vi "Stack_holderwise_total_bd_count_&_duration_2.vi"(0 "Refnum in":T1, 1 "BREAKDOWN_STK_HOLD_ID":i32=1, 2 "condition":string="Where BREAKDOWN_DATE between '%s'and '%s' and BREAKDOWN_STK_HOLD_ID ='%d'  ", 5 "Form Date":timestamp, 7 "Array":string[](array[string]), 9 "To Date":timestamp, 11 "error in (no error)":errorcluster, 12 "STATION_ID_CID_TRIGGER":i32, 13 "Shift":string(combo), 14 "table":string[](array[string])=["STATION_1_LOG_HISTORY", "STATION_2_LOG_HISTORY", "STATION_3_LOG_HISTORY", "STATION_4_LOG_HISTORY", "STATION_5_LOG_HISTORY", "STATION_6_LOG_HISTORY"]) -> (4 "Refnum out":T1, 6 "Count out":string[](array[string]), 10 "appended array":dbl[](array[numeric]), 15 "error out":errorcluster)   [LabVIEW 2017]
uses:
  <vilib>/addons/database/Connection.llb/Conn ObjectReference.ctl
  <vilib>/addons/database/NI_Database_API.lvlib
panel:
  out "Count out 2":string[](array[string])
  out "Table":string[][](array[string])
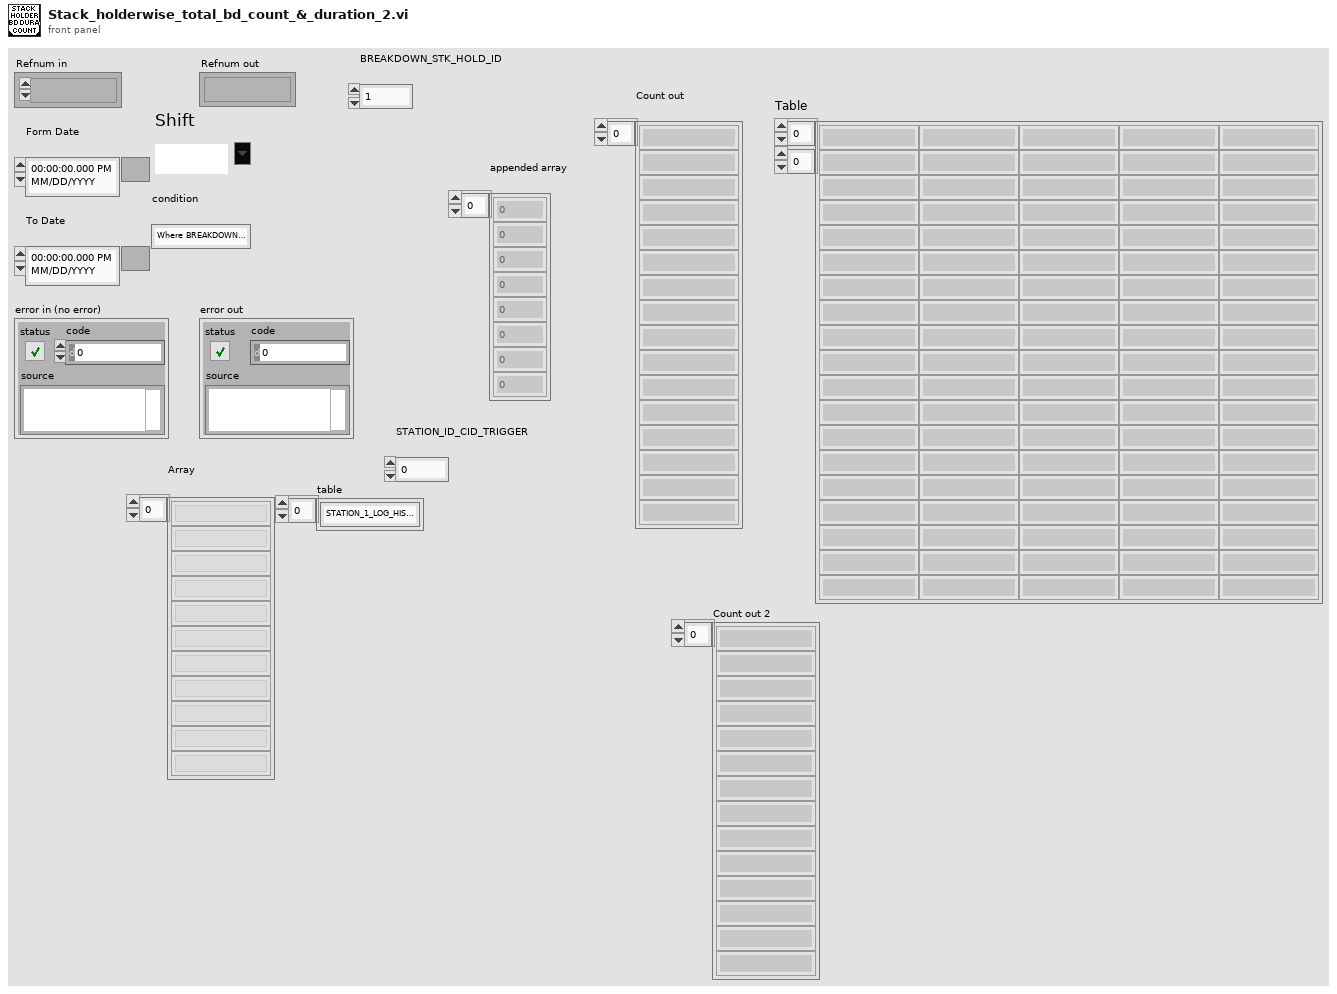
[diagram p1: front panel]
types:
  T1 = typedef "NI_Database_API.lvlib/Conn ObjectReference.ctl" = refnum<k1>
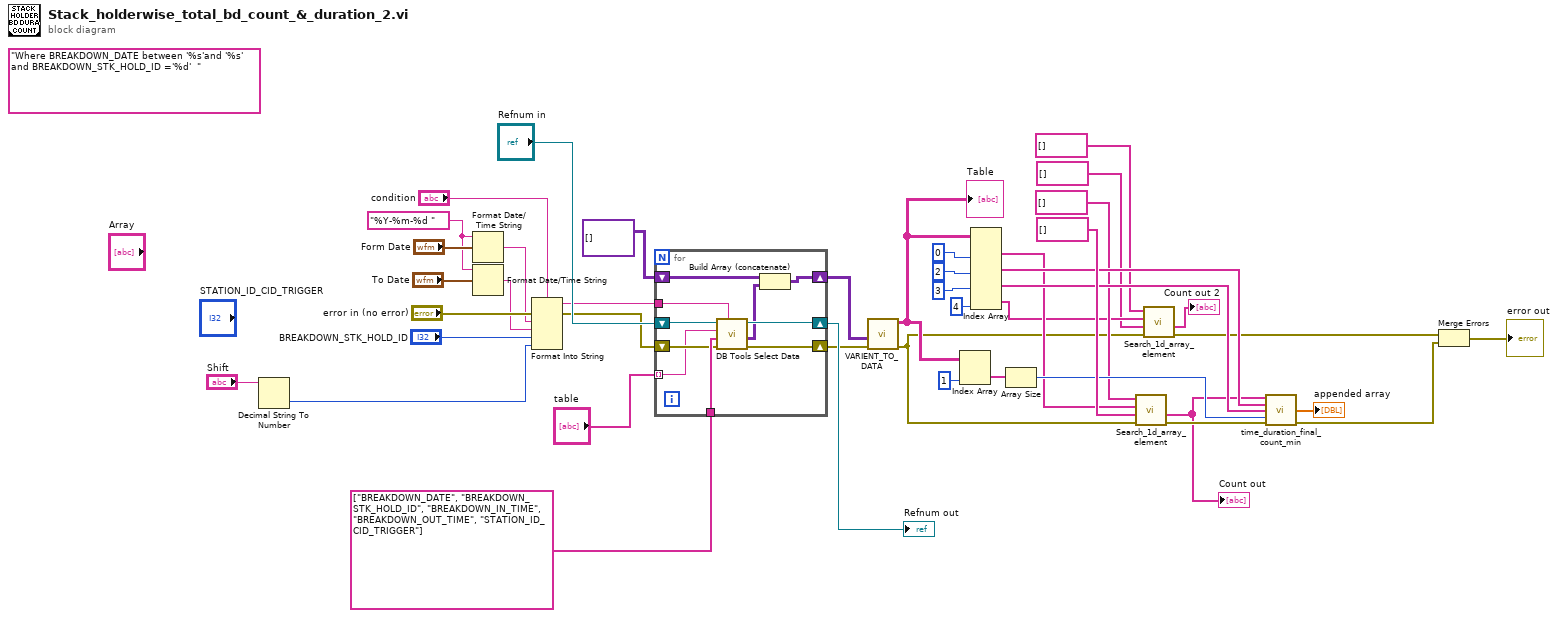
[diagram p0: block diagram]
diagram:
  (unwired) "Where BREAKDOWN_DATE between '%s'and '%s' and BREAKDOWN_STK_HOLD_ID ='%d'  "
  w21 = "%Y-%m-%d " ("time format string (%c)")
  n1 = Decimal String To Number(string="Shift") -> (number=w1:i32)  [unwired: 2 in, 1 out]
  n2 = Format Date/Time String(time format string (%c)=w21, seconds (now)="Form Date") -> (date/time string=w24:string)  [unwired: 1 in]
  n3 = Format Date/Time String(time format string (%c)=w21, seconds (now)="To Date") -> (date/time string=w25:string)  [unwired: 1 in]
  n4 = Format Into String(format string="condition", error in="error in (no error)", w24, w25, "BREAKDOWN_STK_HOLD_ID", w1) -> (resulting string=w17:string, error out=w18:errorcluster)  [unwired: 1 in]
  n5 = for {
    tunnel: string[] ["BREAKDOWN_DATE", "BREAKDOWN_STK_HOLD_ID", "BREAKDOWN_IN_TIME", "BREAKDOWN_OUT_TIME", "STATION_ID_CID_TRIGGER"] -> [w53]
    tunnel: w17 -> [w48]
    shift-right: [w52] -> w28
    shift-left: "Refnum in" -> [w51]
    shift-right: [w50] -> w19
    shift-left: w18 -> [w49]
    shift-right: [w44] -> w20
    shift-left: variant[][] [] ("data") -> [w46]
    tunnel: "table" -> [w47] mode=indexing
    n6 = call <vilib>:"DB Tools Select Data.vi"("condition"=w48, "error in (no error)"=w49, "columns"=w53, "table"=w47, "connection reference"=w51) -> ("error out"=w50:errorcluster, "data"=w45:variant[][], "connection reference out"=w52:T1)  [unwired: 1 in]
    n7 = Build Array (concatenate)(w46, w45) -> (w44:variant[][])
  }
  "Refnum out" <- w28
  n8 = call "VARIENT_TO_DATA.vi"("data"=w20, "error in (no error)"=w19) -> ("Table"=w42:string[][], "error out"=w5:errorcluster)  [unwired: 7 in]
  "Table" <- w42
  n9 = Index Array(array=w42, index (col)=1 ("disabled index (col)")) -> (element=w35:string[])  [unwired: 1 in]
  n10 = Index Array(array=w42, index (col) #1=0 ("disabled index (col)"), index (col) #2=2 ("disabled index (col)"), index (col) #3=3 ("disabled index (col)"), index (col) #4=4 ("disabled index (col)")) -> (element #1=w37:string[], element #2=w39:string[], element #3=w40:string[], element #4=w11:string[])  [unwired: 4 in]
  n11 = Array Size(array=w35) -> (size(s)=w41:i32)
  n12 = call "Search_1d_array_element.vi"("error in (no error)"=w5, "Count in"=string[] [] ("Count"), "BD Date"=w37, "Elements Found in"=string[] [] ("Elements Found")) -> ("error out"=w38:errorcluster, "Count out"=w16:string[])  [unwired: 3 in, 1 out]
  "Count out" <- w16
  n13 = call "Search_1d_array_element.vi"("error in (no error)"=w5, "Count in"=string[] [] ("Count"), "BD Date"=w11, "Elements Found in"=string[] [] ("Elements Found")) -> ("error out"=w4:errorcluster, "Count out"=→"Count out 2":string[])  [unwired: 3 in, 1 out]
  n14 = call "time_duration_final_count_min.vi"("BD Count"=w16, "Intime"=w39, "OutTime"=w40, "bd array size"=w41, "error in (no error)"=w38) -> ("appended array"=→"appended array":dbl[], "error out"=w3:errorcluster)  [unwired: 7 in, 2 out]
  n15 = Merge Errors(w4, w3) -> (→"error out":errorcluster)
